vi "ADC Setup Virtual Channels.vi"(4 "apperture [s] (1.4 us)":dbl=1.4e-06 format="%#_6p", 6 "trigger (immediate)":T1, 7 "voltage ranges [Vpk] (empty: use global default)":dbl[](array[numeric]), 8 "error in":errorcluster, 9 "samples count (100)":i64=100, 10 "fs [Hz] (50k)":dbl=50000.0, 11 "adc session in":T5={"niScope"={"channel cfg"=[], "sessions"=[], "multi cards"=FALSE, "channels"=0, "type"=enum."n/a", "memory [B/chn]"=0, "ext. clock [Hz]"=0.0, "samples count"=0, "use streaming"=FALSE, "proc setup"={"packet size [smpl]"=0, "current timeout [s]"=0.0, "blk2blk timeout [s]"=0.0, "event time"=timestamp(0 s since 1904-01-01), "temp sampl T [s]"=0.0, "data queue"=refnum, "stop notifier"=refnum, "proc ref"=refnum}, "sample width [B]"=0, "ranges [V]"=[], "trigger setup"={"coupling"=1, "level [V]"=0.0, "slope"=0, "mode"=enum."Immediate"}, "fs [Hz]"=0.0, "bitres [bit]"=0}, "3458A"={"channels"=[], "sync unit"={"VISA"="", "type"=enum."Picotest U6200A"}, "awg unit"={"type"=enum."Agilent 331xxA to 332xxA", "VISA"="", "enable 10MHz ref"=FALSE}, "sync mode"=enum."MASTER-SLAVE, MASTER clocked by TIMER", "streaming mode"=FALSE, "idn mode"=enum."Auto", "sampling mode"=enum."DCV", "Ts [s]"=0.0, "sample memory [B]"=0, "proc setup"={"channel id"=0, "packet size [smpl]"=0, "current timeout [s]"=0.0, "blk2blk timeout [s]"=0.0, "event time"=timestamp(0 s since 1904-01-01), "stop notifier"=refnum, "data queues"=[], "proc refs"=[], "bus semaphore"=refnum}, "sample size [B]"=0, "sample count"=0, "aux data"={"channel id"=0, "valid?"=[], "gain [V]"=[], "timestamp [s]"=[], "Ts [s]"=0.0, "abs timestamp"=timestamp(0 s since 1904-01-01), "t [deg C]"=[]}, "ranges [V]"=[], "aperture [s]"=0.0, "LEVEL trigger"={"edge"=enum."POS", "level [V]"=0.0, "coupling"=enum."DC"}, "trigger mode"=enum."AUTO", "measure temp.?"=FALSE, "disp mesages"=[], "shared bus?"=FALSE, "disable display?"=FALSE, "aper mode"=enum."Manual", "aper rules"=[]}, "dsdll"={"dsdll"={"dsdll path"=path "", "dsdll handle"=[], "output devices"=[], "capture devices"=[]}, "channels"=0, "device id"=0, "channel idns"=[], "proc setup"={"packet size [smpl]"=0, "current timeout [s]"=0.0, "blk2blk timeout [s]"=0.0, "event time"=timestamp(0 s since 1904-01-01), "data queue"=refnum, "stop notifier"=refnum, "proc ref"=refnum}, "samples count"=0, "fs [Hz]"=0.0}, "type"=enum."niScope", "channel idn str"=[], "aux instr idn str"=[], "modified?"=FALSE, "simadc"={"channels"=[], "range [V]"=0.0, "Ts step [s]"=0.0, "time [s]"=0.0, "fs [Hz]"=0.0, "count"=0, "smpl offset"=0, "set count"=0, "bit res"=0}, "force rst?"=FALSE, "exit mode"=enum."Immediate reset", "exit dly"=0.0, "exit tmr"=timestamp(0 s since 1904-01-01), "busy?"=FALSE, "accessed?"=FALSE, "QuADC session"={"channel cfg"=[], "sessions"=[], "multi cards"=FALSE, "channels"=0, "type"=enum."n/a", "memory [B/chn]"=0, "ext. clock [Hz]"=0.0, "samples count"=0, "use streaming"=FALSE, "proc setup"={"packet size [smpl]"=0, "current timeout [s]"=0.0, "blk2blk timeout [s]"=0.0, "event time"=timestamp(0 s since 1904-01-01), "temp sampl T [s]"=0.0, "data queue"=refnum, "stop notifier"=refnum, "proc ref"=refnum}, "sample width [B]"=0, "ranges [V]"=[], "trigger setup"={"coupling"=1, "level [V]"=0.0, "slope"=0, "mode"=enum."Immediate"}, "fs [Hz]"=0.0, "bitres [bit]"=0}} {"QuADC session"."trigger setup"."level [V]" format="%.2f"; "QuADC session"."trigger setup"."coupling" items=["AC"=0, "DC"=1, "HF Reject"=3, "LF Reject"=4, "AC Plus HF Reject"=1001]; "QuADC session"."channel cfg"."Range [Vpk]" min=0.0; "QuADC session"."channel cfg"."Channel" min=0; "3458A"."channels"."Range [Vpk]" min=0.0; "niScope"."trigger setup"."level [V]" format="%.2f"; "niScope"."trigger setup"."coupling" items=["AC"=0, "DC"=1, "HF Reject"=3, "LF Reject"=4, "AC Plus HF Reject"=1001]; "niScope"."channel cfg"."Range [Vpk]" min=0.0; "niScope"."channel cfg"."Channel" min=0}) -> (0 "error out":errorcluster, 3 "adc session out":T5={"niScope"={"channel cfg"=[], "sessions"=[], "multi cards"=FALSE, "channels"=0, "type"=enum."n/a", "memory [B/chn]"=0, "ext. clock [Hz]"=0.0, "samples count"=0, "use streaming"=FALSE, "proc setup"={"packet size [smpl]"=0, "current timeout [s]"=0.0, "blk2blk timeout [s]"=0.0, "event time"=timestamp(0 s since 1904-01-01), "temp sampl T [s]"=0.0, "data queue"=refnum, "stop notifier"=refnum, "proc ref"=refnum}, "sample width [B]"=0, "ranges [V]"=[], "trigger setup"={"coupling"=1, "level [V]"=0.0, "slope"=0, "mode"=enum."Immediate"}, "fs [Hz]"=0.0, "bitres [bit]"=0}, "3458A"={"channels"=[], "sync unit"={"VISA"="", "type"=enum."Picotest U6200A"}, "awg unit"={"type"=enum."Agilent 331xxA to 332xxA", "VISA"="", "enable 10MHz ref"=FALSE}, "sync mode"=enum."MASTER-SLAVE, MASTER clocked by TIMER", "streaming mode"=FALSE, "idn mode"=enum."Auto", "sampling mode"=enum."DCV", "Ts [s]"=0.0, "sample memory [B]"=0, "proc setup"={"channel id"=0, "packet size [smpl]"=0, "current timeout [s]"=0.0, "blk2blk timeout [s]"=0.0, "event time"=timestamp(0 s since 1904-01-01), "stop notifier"=refnum, "data queues"=[], "proc refs"=[], "bus semaphore"=refnum}, "sample size [B]"=0, "sample count"=0, "aux data"={"channel id"=0, "valid?"=[], "gain [V]"=[], "timestamp [s]"=[], "Ts [s]"=0.0, "abs timestamp"=timestamp(0 s since 1904-01-01), "t [deg C]"=[]}, "ranges [V]"=[], "aperture [s]"=0.0, "LEVEL trigger"={"edge"=enum."POS", "level [V]"=0.0, "coupling"=enum."DC"}, "trigger mode"=enum."AUTO", "measure temp.?"=FALSE, "disp mesages"=[], "shared bus?"=FALSE, "disable display?"=FALSE, "aper mode"=enum."Manual", "aper rules"=[]}, "dsdll"={"dsdll"={"dsdll path"=path "", "dsdll handle"=[], "output devices"=[], "capture devices"=[]}, "channels"=0, "device id"=0, "channel idns"=[], "proc setup"={"packet size [smpl]"=0, "current timeout [s]"=0.0, "blk2blk timeout [s]"=0.0, "event time"=timestamp(0 s since 1904-01-01), "data queue"=refnum, "stop notifier"=refnum, "proc ref"=refnum}, "samples count"=0, "fs [Hz]"=0.0}, "type"=enum."niScope", "channel idn str"=[], "aux instr idn str"=[], "modified?"=FALSE, "simadc"={"channels"=[], "range [V]"=0.0, "Ts step [s]"=0.0, "time [s]"=0.0, "fs [Hz]"=0.0, "count"=0, "smpl offset"=0, "set count"=0, "bit res"=0}, "force rst?"=FALSE, "exit mode"=enum."Immediate reset", "exit dly"=0.0, "exit tmr"=timestamp(0 s since 1904-01-01), "busy?"=FALSE, "accessed?"=FALSE, "QuADC session"={"channel cfg"=[], "sessions"=[], "multi cards"=FALSE, "channels"=0, "type"=enum."n/a", "memory [B/chn]"=0, "ext. clock [Hz]"=0.0, "samples count"=0, "use streaming"=FALSE, "proc setup"={"packet size [smpl]"=0, "current timeout [s]"=0.0, "blk2blk timeout [s]"=0.0, "event time"=timestamp(0 s since 1904-01-01), "temp sampl T [s]"=0.0, "data queue"=refnum, "stop notifier"=refnum, "proc ref"=refnum}, "sample width [B]"=0, "ranges [V]"=[], "trigger setup"={"coupling"=1, "level [V]"=0.0, "slope"=0, "mode"=enum."Immediate"}, "fs [Hz]"=0.0, "bitres [bit]"=0}} {"QuADC session"."trigger setup"."level [V]" format="%.2f"; "QuADC session"."trigger setup"."coupling" items=["AC"=0, "DC"=1, "HF Reject"=3, "LF Reject"=4, "AC Plus HF Reject"=1001]; "QuADC session"."channel cfg"."Range [Vpk]" min=0.0; "QuADC session"."channel cfg"."Channel" min=0; "3458A"."channels"."Range [Vpk]" min=0.0; "niScope"."trigger setup"."level [V]" format="%.2f"; "niScope"."trigger setup"."coupling" items=["AC"=0, "DC"=1, "HF Reject"=3, "LF Reject"=4, "AC Plus HF Reject"=1001]; "niScope"."channel cfg"."Range [Vpk]" min=0.0; "niScope"."channel cfg"."Channel" min=0})   [LabVIEW 2013]
doc: "Configures ADC virtual channels. Setups all instruments related to the virtual digitizer for digitizing. Voltage ranges input it optional. If not attached VI uses default ranges defined in ADC session. This VI must be called at least once before initiating new record. It is not needed to call it again when multiple records are taken sequentially with the same setup. VI modifies session so do not assign just ADC session in!"
uses:
  ADC Session.ctl
  drivers/niScope/niScope Session.ctl
  drivers/niScope/niScope Virtual Channel Config.ctl
  drivers/niScope/niScope Virtual Channel Mode.ctl
  drivers/niScope/niScope Virtual Channel Input Z.ctl
  drivers/niScope/niScope Virtual Channel Coupling.ctl
  drivers/niScope/niScope Type.ctl
  drivers/niScope/niScope Digitizing Process Options.ctl
  drivers/niScope/niScope Data Packet.ctl
  drivers/niScope/niScope Trigger Setup.ctl
  <instrlib>/niScope/Controls/niScope trigger coupling.ctl
  <instrlib>/niScope/Controls/niScope trigger slope.ctl
  drivers/DMM/3458A Digitizer Session.ctl
  drivers/DMM/3458A Virtual Channel Config.ctl
  drivers/Counter/Counter Session.ctl
  drivers/Counter/Counter Type.ctl
  drivers/AWG/AWG Session.ctl
  drivers/AWG/AWG Type.ctl
  drivers/DMM/3458A Sync Mode.ctl
  drivers/DMM/3458A Idn Mode.ctl
  drivers/DMM/3458A Digitizing Low Levels/Configure/Sampling Mode.ctl
  drivers/DMM/3458A Digitizing Process Options.ctl
  drivers/DMM/3458A Data Packet.ctl
  drivers/DMM/3458A Aux Record Data.ctl
  drivers/DMM/3458A Digitizing Low Levels/Configure/Level Setup.ctl
  drivers/DMM/3458A Digitizing Low Levels/Configure/First Sample Trigger.ctl
  drivers/DMM/3458A Aperture Selection Mode.ctl
  drivers/dsdll/DSDLL Session.ctl
  drivers/dsdll/dsdll.lvlibp/dsdll_instance.ctl
  drivers/dsdll/dsdll.lvlibp/dsdll_device_record.ctl
  drivers/dsdll/DSDLL Process Config.ctl
  drivers/dsdll/DSDLL Data Packet.ctl
  ADC Type.ctl
  drivers/simulated_adc/SimAdc Config.ctl
  drivers/simulated_adc/SimAdc Channel Cfg.ctl
  ADC On Close Action.ctl
  drivers/Quatsch_driver/QuADCDriver/QuADC Session.ctl
  drivers/Quatsch_driver/QuADCDriver/QuADC Virtual Channel Config.ctl
  drivers/Quatsch_driver/QuADCDriver/QuADC Virtual Channel Mode.ctl
  drivers/Quatsch_driver/QuADCDriver/QuADC Virtual Channel Input Z.ctl
  drivers/Quatsch_driver/QuADCDriver/QuADC Virtual Channel Coupling.ctl
  drivers/Quatsch_driver/QuADCDriver/QuADC Type.ctl
  drivers/Quatsch_driver/QuADCDriver/QuADC Digitizing Process Options.ctl
  drivers/Quatsch_driver/QuADCDriver/QuADC Data Packet.ctl
  drivers/Quatsch_driver/QuADCDriver/QuADC Trigger Setup.ctl
  ADC Trig Config.ctl
  ADC Trig Mode Source.ctl
  ADC Trig Coupling.ctl
  ADC Trig Slope.ctl
  <vilib>/Utility/error.llb/Error Cluster From Error Code.vi
  <vilib>/ErrorRing/Error Ring.xnode
  drivers/niScope/niScope Virtual Digitizer.lvlib
  drivers/DMM/3458A Virtual Digitizer.lvlib
  drivers/DMM/3458A Digitizing Low Levels/3458A Digitizing Low Levels.lvlib
  drivers/dsdll/DSDLL Virtual Digitizer.lvlib
  drivers/Quatsch_driver/QuADCDriver/QuADC Virtual Digitizer.lvlib
  drivers/Counter/Counter.lvlib
  drivers/AWG/AWG.lvlib
  drivers/dsdll/dsdll.lvlibp
panel:
  # "IP Address"
  # "."
  # "."
  # "."
  # ":"
  # "IP Address"
  # "."
  # "."
  # "."
  # ":"
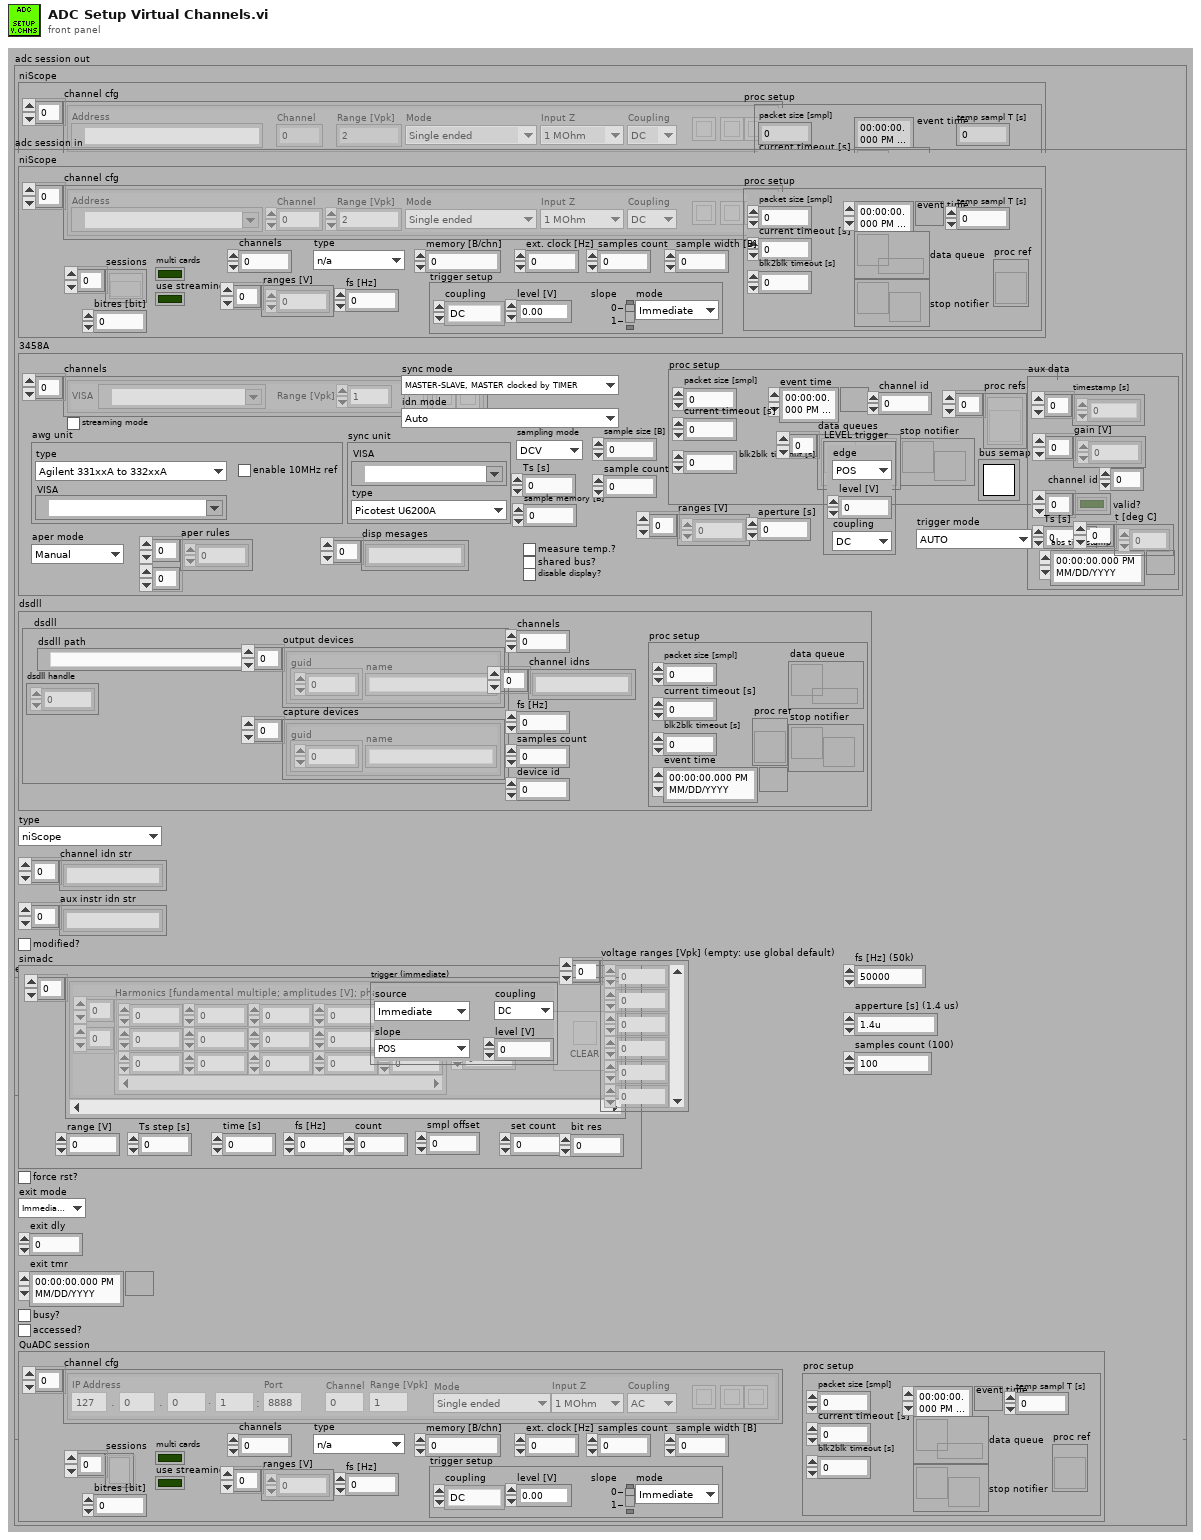
[diagram p1: front panel]
types:
  T1 = typedef "ADC Trig Config.ctl" = cluster{"source":T2, "level [V]":dbl, "coupling":T3, "slope":T4}
  T2 = typedef "ADC Trig Mode Source.ctl" = enum16{"Immediate", "External", "Level"}
  T3 = typedef "ADC Trig Coupling.ctl" = enum16{"DC", "AC"}
  T4 = typedef "ADC Trig Slope.ctl" = enum16{"POS", "NEG"}
  T5 = typedef "ADC Session.ctl" = cluster{"niScope":T6, "3458A":T16, "dsdll":T31, "type":T35, "channel idn str":string[], "aux instr idn str":string[], "modified?":bool, "simadc":T36, "force rst?":bool, "exit mode":T38, "exit dly":dbl, "exit tmr":timestamp, "busy?":bool, "accessed?":bool, "QuADC session":T39}
  T6 = typedef "niScope Virtual Digitizer.lvlib/niScope Session.ctl" = cluster{"channel cfg":T7[], "sessions":refnum<k20>[], "multi cards":bool, "channels":i32, "type":T11, "memory [B/chn]":i32, "ext. clock [Hz]":dbl, "samples count":i64, "use streaming":bool, "proc setup":T12, "sample width [B]":i32, "ranges [V]":dbl[], "trigger setup":T13, "fs [Hz]":dbl, "bitres [bit]":i32}
  T7 = typedef "niScope Virtual Digitizer.lvlib/niScope Virtual Channel Config.ctl" = cluster{"Address":refnum<k15>, "Channel":i32, "Mode":T8, "Input Z":T9, "Coupling":T10, "Range [Vpk]":dbl, "btn clr":bool, "btn up":bool, "btn down":bool}
  T8 = typedef "niScope Virtual Digitizer.lvlib/niScope Virtual Channel Mode.ctl" = enum16{"Single ended", "Unbal. differential", "Differential"}
  T9 = typedef "niScope Virtual Digitizer.lvlib/niScope Virtual Channel Input Z.ctl" = enum16{"1 MOhm", "50 Ohm"}
  T10 = typedef "niScope Virtual Digitizer.lvlib/niScope Virtual Channel Coupling.ctl" = enum16{"AC", "DC", "GND"}
  T11 = typedef "niScope Virtual Digitizer.lvlib/niScope Type.ctl" = enum16{"n/a", "5922"}
  T12 = typedef "niScope Virtual Digitizer.lvlib/niScope Digitizing Process Options.ctl" = cluster{"packet size [smpl]":i64, "current timeout [s]":dbl, "blk2blk timeout [s]":dbl, "event time":timestamp, "temp sampl T [s]":dbl, "data queue":refnum<queue>, "stop notifier":refnum<notifier>, "proc ref":refnum<vi>}
  T13 = typedef "niScope Virtual Digitizer.lvlib/niScope Trigger Setup.ctl" = cluster{"coupling":T14, "level [V]":dbl, "slope":T15, "mode":enum16{"Immediate", "External", "Level"}}
  T14 = typedef "niScope trigger coupling.ctl" = u16
  T15 = typedef "niScope trigger slope.ctl" = i32
  T16 = typedef "3458A Virtual Digitizer.lvlib/3458A Digitizer Session.ctl" = cluster{"channels":T17[], "sync unit":T18, "awg unit":T20, "sync mode":T22, "streaming mode":bool, "idn mode":T23, "sampling mode":T24, "Ts [s]":dbl, "sample memory [B]":i32, "proc setup":T25, "sample size [B]":i32, "sample count":i32, "aux data":T27, "ranges [V]":dbl[], "aperture [s]":dbl, "LEVEL trigger":T28, "trigger mode":T29, "measure temp.?":bool, "disp mesages":string[], "shared bus?":bool, "disable display?":bool, "aper mode":T30, "aper rules":dbl[][]}
  T17 = typedef "3458A Virtual Digitizer.lvlib/3458A Virtual Channel Config.ctl" = cluster{"VISA":refnum<visa-resource-name>, "Range [Vpk]":dbl, "btn clr":bool, "btn up":bool, "btn down":bool}
  T18 = typedef "Counter.lvlib/Counter Session.ctl" = cluster{"VISA":refnum<visa-resource-name>, "type":T19}
  T19 = typedef "Counter.lvlib/Counter Type.ctl" = enum16{"Picotest U6200A", "dummy"}
  T20 = typedef "AWG.lvlib/AWG Session.ctl" = cluster{"type":T21, "VISA":refnum<visa-resource-name>, "enable 10MHz ref":bool}
  T21 = typedef "AWG.lvlib/AWG Type.ctl" = enum16{"Agilent 331xxA to 332xxA", "Agilent 335xxA to 336xxA", "Tektronix AFG3101C", "dummy"}
  T22 = typedef "3458A Virtual Digitizer.lvlib/3458A Sync Mode.ctl" = enum16{"MASTER-SLAVE, MASTER clocked by TIMER", "MASTER-SLAVE, MASTER clocked by AWG", "ALL clocked by AWG", "MASTER-SLAVE, ALL clocked by TIMER", "ALL clocked by AWG with DFLL"}
  T23 = typedef "3458A Virtual Digitizer.lvlib/3458A Idn Mode.ctl" = enum16{"Auto", "Sequential (chn A, chn B, ...)", "From calibration string"}
  T24 = typedef "3458A Virtual Digitizer.lvlib/3458A Digitizing Low Levels.lvlib/Sampling Mode.ctl" = enum16{"DCV", "DSDC", "DSAC"}
  T25 = typedef "3458A Virtual Digitizer.lvlib/3458A Digitizing Process Options.ctl" = cluster{"channel id":i32, "packet size [smpl]":i32, "current timeout [s]":dbl, "blk2blk timeout [s]":dbl, "event time":timestamp, "stop notifier":refnum<notifier>, "data queues":refnum<queue>[], "proc refs":refnum<vi>[], "bus semaphore":T26}
  T26 = typedef "Semaphore RefNum" = refnum<k1>
  T27 = typedef "3458A Virtual Digitizer.lvlib/3458A Aux Record Data.ctl" = cluster{"channel id":i32, "valid?":bool[], "gain [V]":dbl[], "timestamp [s]":dbl[], "Ts [s]":dbl, "abs timestamp":timestamp, "t [deg C]":dbl[]}
  T28 = typedef "3458A Virtual Digitizer.lvlib/3458A Digitizing Low Levels.lvlib/Level Setup.ctl" = cluster{"edge":enum16{"POS", "NEG"}, "level [V]":dbl, "coupling":enum16{"DC", "AC"}}
  T29 = typedef "3458A Virtual Digitizer.lvlib/3458A Digitizing Low Levels.lvlib/First Sample Trigger.ctl" = enum16{"AUTO", "EXT", "SYN", "SGL", "HOLD", "LEVEL"}
  T30 = typedef "3458A Virtual Digitizer.lvlib/3458A Aperture Selection Mode.ctl" = enum16{"Manual", "Maximum", "Table"}
  T31 = typedef "DSDLL Virtual Digitizer.lvlib/DSDLL Session.ctl" = cluster{"dsdll":T32, "channels":i32, "device id":i32, "channel idns":string[], "proc setup":T34, "samples count":i32, "fs [Hz]":dbl}
  T32 = typedef "dsdll.lvlibp/dsdll_instance.ctl" = cluster{"dsdll path":path, "dsdll handle":u8[], "output devices":T33[], "capture devices":T33[]}
  T33 = typedef "dsdll.lvlibp/dsdll_device_record.ctl" = cluster{"guid":u8[], "name":string}
  T34 = typedef "DSDLL Virtual Digitizer.lvlib/DSDLL Process Config.ctl" = cluster{"packet size [smpl]":i32, "current timeout [s]":dbl, "blk2blk timeout [s]":dbl, "event time":timestamp, "data queue":refnum<queue>, "stop notifier":refnum<notifier>, "proc ref":refnum<vi>}
  T35 = typedef "ADC Type.ctl" = enum16{"niScope", "3458A", "DirectSound DLL", "dummy", "QuADC"}
  T36 = typedef "SimAdc Config.ctl" = cluster{"channels":T37[], "range [V]":dbl, "Ts step [s]":dbl, "time [s]":dbl, "fs [Hz]":dbl, "count":i64, "smpl offset":i64, "set count":i64, "bit res":i32}
  T37 = typedef "SimAdc Channel Cfg.ctl" = cluster{"harmonics":dbl[][], "btn clear":bool, "noise":dbl, "fundamental [Hz]":dbl}
  T38 = typedef "ADC On Close Action.ctl" = enum16{"Immediate reset", "Delayed reset"}
  T39 = typedef "QuADC Virtual Digitizer.lvlib/QuADC Session.ctl" = cluster{"channel cfg":T40[], "sessions":refnum<k5>[], "multi cards":bool, "channels":i32, "type":T44, "memory [B/chn]":i32, "ext. clock [Hz]":dbl, "samples count":i64, "use streaming":bool, "proc setup":T45, "sample width [B]":i32, "ranges [V]":dbl[], "trigger setup":T46, "fs [Hz]":dbl, "bitres [bit]":i32}
  T40 = typedef "QuADC Virtual Digitizer.lvlib/QuADC Virtual Channel Config.ctl" = cluster{"Channel":i32, "Mode":T41, "Input Z":T42, "Coupling":T43, "Range [Vpk]":dbl, "btn clr":bool, "btn up":bool, "btn down":bool, "IP address A":u8, "IP address B":u8, "IP address C":u8, "IP address D":u8, "Port":u16}
  T41 = typedef "QuADC Virtual Digitizer.lvlib/QuADC Virtual Channel Mode.ctl" = enum16{"Single ended", "Unbal. differential", "Differential"}
  T42 = typedef "QuADC Virtual Digitizer.lvlib/QuADC Virtual Channel Input Z.ctl" = enum16{"1 MOhm", "50 Ohm"}
  T43 = typedef "QuADC Virtual Digitizer.lvlib/QuADC Virtual Channel Coupling.ctl" = enum16{"AC", "DC", "GND"}
  T44 = typedef "QuADC Virtual Digitizer.lvlib/QuADC Type.ctl" = enum16{"n/a", "v1"}
  T45 = typedef "QuADC Virtual Digitizer.lvlib/QuADC Digitizing Process Options.ctl" = cluster{"packet size [smpl]":i64, "current timeout [s]":dbl, "blk2blk timeout [s]":dbl, "event time":timestamp, "temp sampl T [s]":dbl, "data queue":refnum<queue>, "stop notifier":refnum<notifier>, "proc ref":refnum<vi>}
  T46 = typedef "QuADC Virtual Digitizer.lvlib/QuADC Trigger Setup.ctl" = cluster{"coupling":T14, "level [V]":dbl, "slope":T15, "mode":enum16{"Immediate", "External", "Level"}}
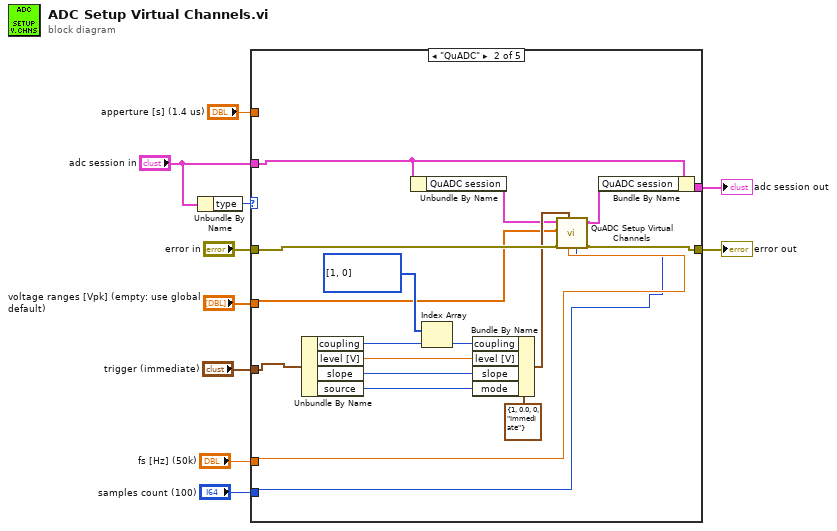
[diagram p0: block diagram]
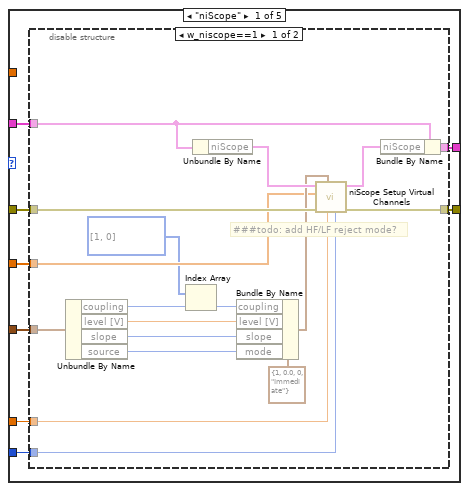
[diagram p2: hidden frame]
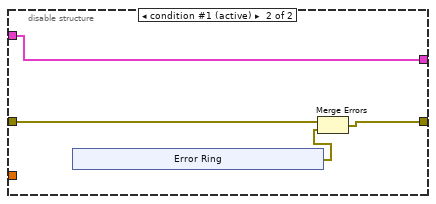
[diagram p3: hidden frame]
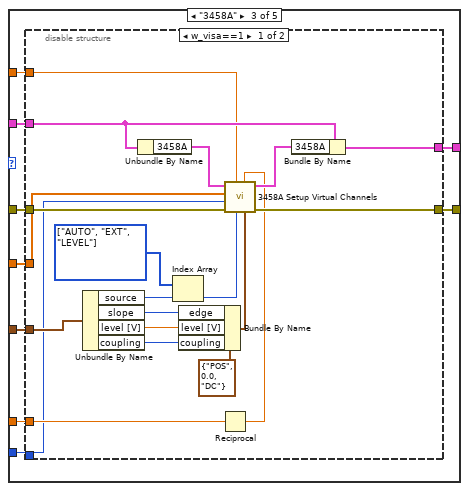
[diagram p4: hidden frame]
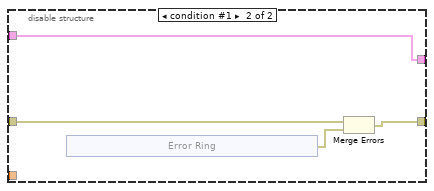
[diagram p5: hidden frame]
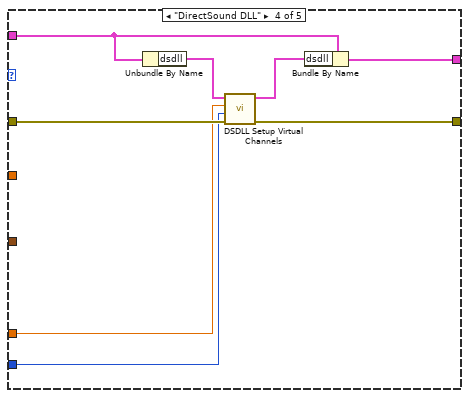
[diagram p6: hidden frame]
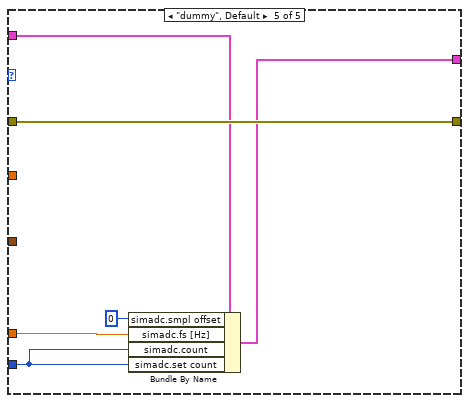
[diagram p7: hidden frame]
diagram:
  n1 = Unbundle By Name("adc session in") -> ("type"=w10:T35)
  n2 = case shown="\"QuADC\"" w10 {
    tunnel: "error in" -> [w18 w54 w72 w109 w115]
    tunnel: "adc session in" -> [w17 w56 w71 w107 w113]
    tunnel: [w16 w46 w70 w106 w112] -> w7
    tunnel: [w15 w55 w69 w105 w115] -> w6
    tunnel: "trigger (immediate)" -> [w14 w49 w68 _ _]
    tunnel: "voltage ranges [Vpk] (empty: use global default)" -> [w13 w50 w67 _ _]
    tunnel: "fs [Hz] (50k)" -> [w12 w48 w66 w103 w114]
    tunnel: "apperture [s] (1.4 us)" -> [_ _ w65 _ _]
    tunnel: "samples count (100)" -> [w11 w47 w64 w102 w111]
    frame "niScope" {
      n3 = disable-structure shown="w_niscope==1" {
        disable-tunnel: w18 -> [w36 w39]
        disable-tunnel: w17 -> [w34 w37]
        disable-tunnel: [w32 w37] -> w16
        disable-tunnel: [w31 w38] -> w15
        disable-tunnel: w14 -> [w28 _]
        disable-tunnel: w13 -> [w24 _]
        disable-tunnel: w12 -> [w23 _]
        disable-tunnel: w11 -> [w22 _]
        frame condition #0 {
          w21 = T14[] [1, 0] items=["AC"=0, "DC"=1, "HF Reject"=3, "LF Reject"=4, "AC Plus HF Reject"=1001]
          # "###todo: add HF/LF reject mode?"
          n4 = Unbundle By Name(w28) -> ("coupling"=w19:T3, "level [V]"=w25:dbl, "slope"=w26:T4, "source"=w27:T2)
          n5 = Index Array(array=w21, index=w19) -> (element=w20:T14)
          n6 = Unbundle By Name(w34) -> ("niScope"=w35:T6)
          n7 = Bundle By Name(cluster=T13 {"coupling"=1, "level [V]"=0.0, "slope"=0, "mode"=enum."Immediate"} ("trigger setup (Immediate)"), "coupling"=w20, "level [V]"=w25, "slope"=w26, "mode"=w27) -> (w29:T13)
          n8 = call "niScope Setup Virtual Channels.vi"("samples count"=w22, "fs [Hz]"=w23, "trigger setup (Immediate)"=w29, "error in"=w36, "voltage ranges [Vpk] (empty: use global default)"=w24, "niScope in"=w35) -> ("error out"=w31:errorcluster, "niScope out"=w33:T6)  [unwired: 4 in]
          n9 = Bundle By Name(cluster=w34, "niScope"=w33) -> (w32:T5)
        }
        frame condition #1 (active) {
          n10 = xnode "Error Ring"() -> ("error out"=w40:errorcluster)
          n11 = Merge Errors(w39, w40) -> (w38:errorcluster)
        }
      }
    }
    frame "QuADC" {
      w59 = T14[] [1, 0] items=["AC"=0, "DC"=1, "HF Reject"=3, "LF Reject"=4, "AC Plus HF Reject"=1001]
      n12 = Unbundle By Name(w49) -> ("coupling"=w57:T3, "level [V]"=w60:dbl, "slope"=w61:T4, "source"=w62:T2)
      n13 = Unbundle By Name(w56) -> ("QuADC session"=w51:T39)
      n14 = Index Array(array=w59, index=w57) -> (element=w58:T14)
      n15 = Bundle By Name(cluster=T13 {"coupling"=1, "level [V]"=0.0, "slope"=0, "mode"=enum."Immediate"} ("trigger setup (Immediate)"), "coupling"=w58, "level [V]"=w60, "slope"=w61, "mode"=w62) -> (w53:T13)
      n16 = call "QuADC Setup Virtual Channels.vi"("samples count"=w47, "fs [Hz]"=w48, "trigger setup (Immediate)"=w53, "error in"=w54, "voltage ranges [Vpk] (empty: use global default)"=w50, "QuADC in"=w51) -> ("error out"=w55:errorcluster, "QuADC out"=w52:T39)  [unwired: 4 in]
      n17 = Bundle By Name(cluster=w56, "QuADC session"=w52) -> (w46:T5)
    }
    frame "3458A" {
      n18 = disable-structure shown="w_visa==1" {
        disable-tunnel: w72 -> [w92 w95]
        disable-tunnel: w71 -> [w90 w93]
        disable-tunnel: [w89 w93] -> w70
        disable-tunnel: [w88 w94] -> w69
        disable-tunnel: w68 -> [w86 _]
        disable-tunnel: w67 -> [w79 _]
        disable-tunnel: w66 -> [w78 _]
        disable-tunnel: w65 -> [w76 _]
        disable-tunnel: w64 -> [w75 _]
        frame condition #0 (active) {
          w85 = T29[] [enum."AUTO", enum."EXT", enum."LEVEL"] items=["AUTO", "EXT", "SYN", "SGL", "HOLD", "LEVEL"]
          n19 = Unbundle By Name(w86) -> ("source"=w84:T2, "slope"=w74:T4, "level [V]"=w80:dbl, "coupling"=w73:T3)
          n20 = Unbundle By Name(w90) -> ("3458A"=w87:T16)
          n21 = Index Array(array=w85, index=w84) -> (element=w83:T29)
          n22 = Bundle By Name(cluster=T28 {"edge"=enum."POS", "level [V]"=0.0, "coupling"=enum."DC"} ("LEVEL trigger"), "edge"=w74, "level [V]"=w80, "coupling"=w73) -> (w82:T28)
          n23 = Reciprocal(x=w78) -> (1/x=w77:dbl)
          n24 = call "3458A Setup Virtual Channels.vi"("LEVEL trigger"=w82, "sample period [s] (1 ms)"=w77, "TRIG source (AUTO)"=w83, "apperture [s] (1.4 us)"=w76, "error in"=w92, "samples count (100)"=w75, "voltage ranges [Vpk] (empty: use global default)"=w79, "digitizer in"=w87) -> ("error out"=w88:errorcluster, "digitizer out"=w91:T16)  [unwired: 2 in]
          n25 = Bundle By Name(cluster=w90, "3458A"=w91) -> (w89:T5)
        }
        frame condition #1 {
          n26 = xnode "Error Ring"() -> ("error out"=w96:errorcluster)
          n27 = Merge Errors(w95, w96) -> (w94:errorcluster)
        }
      }
    }
    frame "DirectSound DLL" {
      n28 = Unbundle By Name(w107) -> ("dsdll"=w104:T31)
      n29 = call "DSDLL Setup Virtual Channels.vi"("error in"=w109, "samples count"=w102, "sample rate [Hz]"=w103, "dsdll session"=w104) -> ("error out"=w105:errorcluster, "dsdll session out"=w108:T31)  [unwired: 6 in]
      n30 = Bundle By Name(cluster=w107, "dsdll"=w108) -> (w106:T5)
    }
    frame "dummy", Default {
      n31 = Bundle By Name(cluster=w113, "simadc.smpl offset"=i64 0, "simadc.fs [Hz]"=w114, "simadc.count"=w111, "simadc.set count"=w111) -> (w112:T5)
    }
  }
  "error out" <- w6
  "adc session out" <- w7
